vi "4.1.vi"(10 "input variable":i32) -> (2 "output variable":i32)   [LabVIEW 2013]
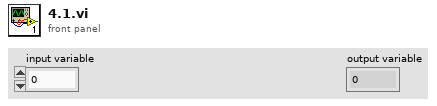
[diagram p1: front panel]
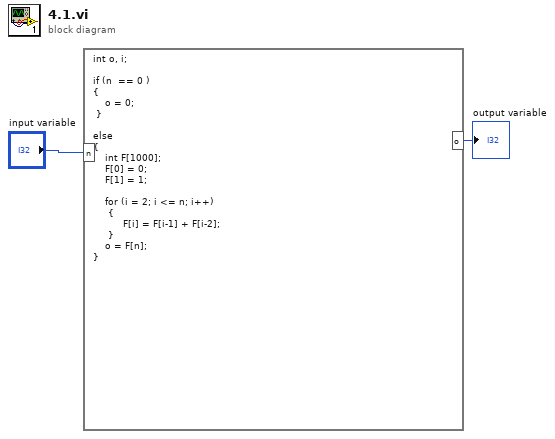
[diagram p0: block diagram]
diagram:
  n1 = formula code="int o, i;\n\nif (n  == 0 ) \n{ \n    o = 0;\n }\n\nelse \n{\n    int F[1000];\n    F[0] = 0;\n    F[1] = 1;\n\n    for (i = 2; i <= n; i++)\n     {\n          F[i] = F[i-1] + F[i-2];     \n     }\n    o = F[n]; \n}"("n"="input variable") -> ("o"=→"output variable":i32)
